vi "New.vi"(8 "error in (no error)":errorcluster, 11 "reference in":refnum<class "FrameworkSubTestSuite.lvclass">) -> (0 "error out":errorcluster, 3 "reference out":refnum<class "FrameworkSubTestSuite.lvclass">)   [LabVIEW 2013, in "FrameworkSubTestSuite.lvclass"]
uses:
  FrameworkSubTestSuite.lvclass
  DoNotWaitOnTestComplete/DoNotWaitOnTestComplete.lvclass
  Classes/TestSuite/TestSuite.lvclass
  Classes/TestCase/TestCase.lvclass
  Classes/TestLoader/TestLoader.lvclass
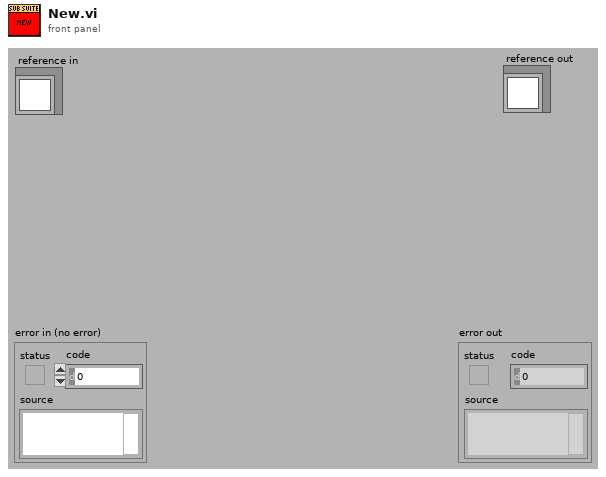
[diagram p1: front panel]
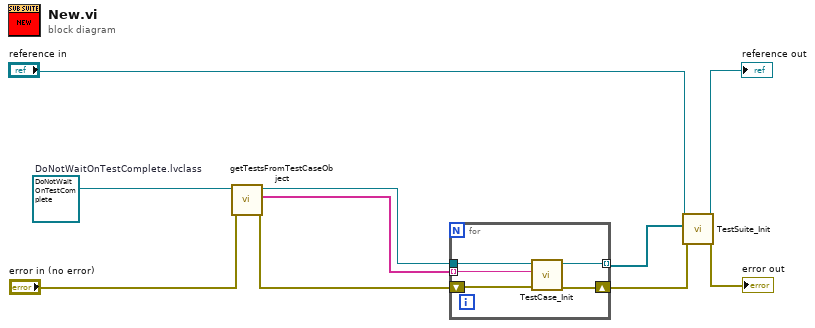
[diagram p0: block diagram]
diagram:
  w2 = refnum<class "DoNotWaitOnTestComplete.lvclass"> refnum  # DoNotWaitOnTestComplete.lvclass
  n1 = call "getTestsFromTestCaseObject.vi"("error in"="error in (no error)", "Test in"=w2) -> ("error out"=w4:errorcluster, "Test Method Names"=w3:string[], "Test out"=w1:refnum<class "DoNotWaitOnTestComplete.lvclass">)  [unwired: 7 in]
  n2 = for {
    shift-right: [w14] -> w8
    shift-left: w4 -> [w15]
    tunnel: [w13] -> w7 mode=indexing
    tunnel: w3 -> [w12] mode=indexing
    tunnel: w1 -> [w11]
    n3 = call "TestCase_Init.vi"("error in (no error)"=w15, "methodName (\"runTest\")"=w12, "TestCase in"=w11) -> ("error out"=w14:errorcluster, "TestCase out"=w13:refnum<class "DoNotWaitOnTestComplete.lvclass">)  [unwired: 7 in]
  }
  n4 = call "TestSuite_Init.vi"("error in (no error)"=w8, "tests (none)"=w7, "TestSuite in"="reference in") -> ("error out"=→"error out":errorcluster, "TestSuite out"=→"reference out":refnum<class "FrameworkSubTestSuite.lvclass">)  [unwired: 7 in]
